vi "Vendor ID.vi"(4 "node-ID":u8 format="%x", 5 "error in":errorcluster, 8 "interface object in":refnum<k20>) -> (0 "error out":errorcluster, 1 "Vendor ID":u32 format="%x", 2 "completion code":u32 format="%.0x", 3 "interface object out":refnum<k20>)   [LabVIEW 2016]
uses:
  <vilib>/CANopenLib/CANOPEN.llb/CANopen SDO Create.vi
  <vilib>/CANopenLib/CANOPEN.llb/CANopen SDO Close.vi
panel:
  out "description":string
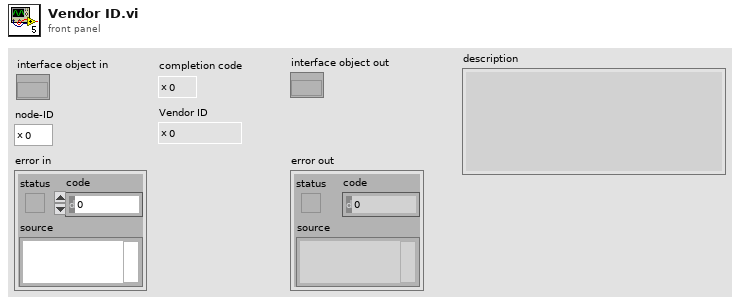
[diagram p1: front panel]
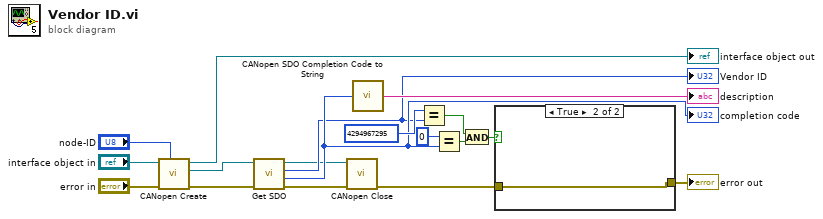
[diagram p0: block diagram]
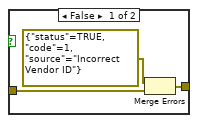
[diagram p2: hidden frame]
diagram:
  n1 = call-poly <vilib>:"CANopen Create.vi"("node-ID"="node-ID", "error in (no error)"="error in", "interface object in"="interface object in") -> ("error out"=w2:errorcluster, "SDO object out"=w1:refnum<k20>, "interface object out"=→"interface object out":refnum<k20>)  [unwired: 6 in]
  n2 = call-poly "Get SDO.vi"("error in (no error)"=w2, "SDO object in"=w1) -> ("error out"=w4:errorcluster, "completion code"=w7:u32, "U32 data"=w6:u32, "SDO object out"=w5:refnum<k20>)  [unwired: 6 in]
  "Vendor ID" <- w6
  "completion code" <- w7
  n3 = call-poly <vilib>:"CANopen Close.vi"("error in (no error)"=w4, "SDO object in"=w5) -> ("error out"=w9:errorcluster)  [unwired: 9 in]
  n4 = call <vilib>:"CANopen SDO Completion Code to String.vi"("SDO completion code"=w7) -> ("description"=→"description":string)
  n5 = Equal?(x=u32 4294967295 ("y"), y=w6) -> (x = y?=w15:bool)
  n6 = Equal?(x=u32 0 ("y"), y=w7) -> (x = y?=w14:bool)
  n7 = And(x=w15, y=w14) -> (x .and. y?=w12:bool)
  n8 = case shown="True" w12 {
    tunnel: w9 -> [w20 w22]
    tunnel: [w19 w22] -> w13
    frame False {
      n9 = Merge Errors(errorcluster {"status"=TRUE, "code"=1, "source"="Incorrect Vendor ID"} ("error constant"), w20) -> (w19:errorcluster)
    }
    frame True {
    }
  }
  "error out" <- w13
